vi "Message Window update.vi"(9 "String Control":string="Current Consumption Test   ", 10 "Previous":string, 11 "Stat":string) -> (3 "String":string)   [LabVIEW 2018, in "LED Control Module.lvlib"]
uses:
  LED Control Module.lvlib
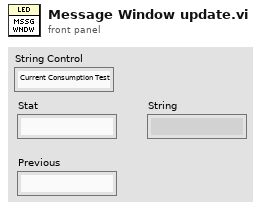
[diagram p1: front panel]
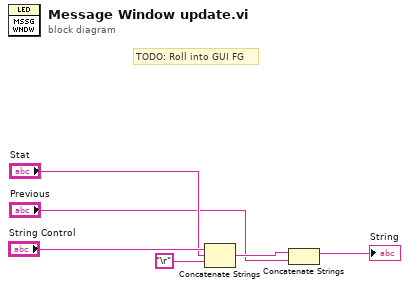
[diagram p0: block diagram]
diagram:
  # "TODO: Roll into GUI FG"
  n1 = Concatenate Strings("String Control", "Stat", "\r") -> (w4:string)
  n2 = Concatenate Strings(w4, "Previous") -> (→"String":string)
